vi "PDP MagRemote Message.vi"   [LabVIEW 2010]
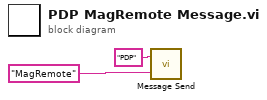
[diagram p0: block diagram]
diagram:
  n1 = call "Message Send.vi"("Message"="MagRemote", "Destination"="PDP") -> ()
